vi "fillDataArray.vi"(6 "Data":dbl[][](array[numeric]), 8 "error in (no error)":errorcluster, 9 "fill number":i32[](array[numeric]), 10 "position":i32[](array[numeric]), 11 "SoundAO in":refnum<class "SoundAO.lvclass">) -> (0 "error out":errorcluster, 2 "transformedData":dbl[][](array[numeric]), 3 "SoundAO out":refnum<class "SoundAO.lvclass">)   [LabVIEW 2011, in "Hardware.lvlib" / "Channels.lvlib" / "SoundAO.lvclass"]
uses:
  SoundAO.lvclass
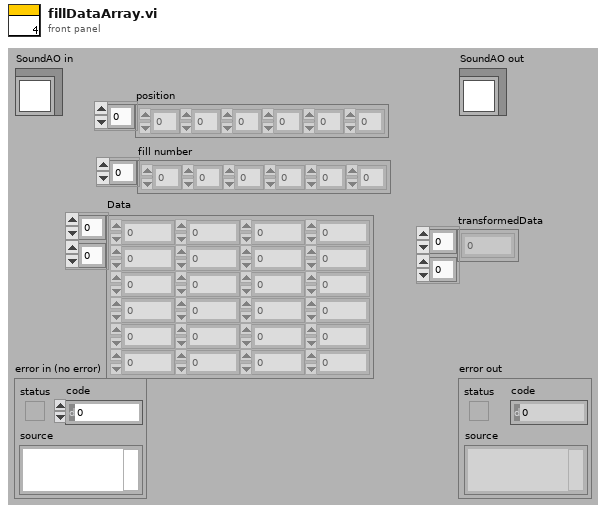
[diagram p1: front panel]
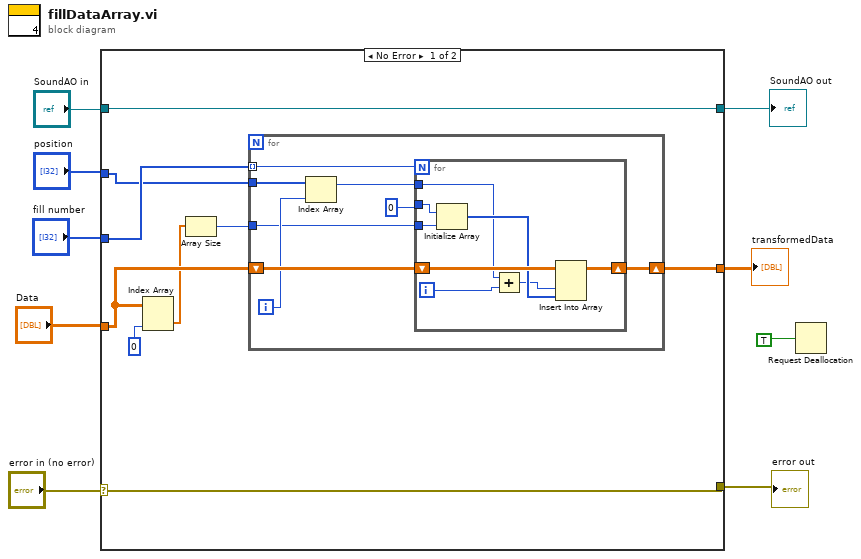
[diagram p0: block diagram]
diagram:
  n1 = case shown="No Error" "error in (no error)" {
    selector: "error in (no error)" -> [w14 w36]
    tunnel: [w14 w36] -> w7
    tunnel: [w16 w35] -> w8
    tunnel: "SoundAO in" -> [w16 w35]
    tunnel: "position" -> [w17 _]
    tunnel: "fill number" -> [w18 _]
    tunnel: "Data" -> [w12 _]
    tunnel: [w13 _] -> w2
    frame No Error {
      n2 = Index Array(array=w12, index (col)=0) -> (element=w10:dbl[])  [unwired: 1 in]
      n3 = Array Size(array=w10) -> (size(s)=w15:i32)
      n4 = for {
        tunnel: w18 -> [w23] mode=indexing
        shift-right: [w24] -> w13
        shift-left: w12 -> [w25]
        tunnel: w17 -> [w22]
        tunnel: w15 -> [w19]
        i -> [w21]
        n5 = Index Array(array=w22, index=w21) -> (element=w20:i32)
        n6 = for {
          N: w23 -> [_]
          tunnel: 0 -> [w34]
          shift-right: [w31] -> w24
          shift-left: w25 -> [w33]
          tunnel: w20 -> [w29]
          tunnel: w19 -> [w27]
          i -> [w30]
          n7 = Initialize Array(w34, w27) -> (w32:i32[])
          n8 = Add(x=w29, y=w30) -> (x+y=w28:i32)
          n9 = Insert Into Array(array=w33, index (col)=w28, new element=w32) -> (w31:dbl[][])  [unwired: 1 in]
        }
      }
    }
    frame Error {
    }
  }
  "error out" <- w7
  "SoundAO out" <- w8
  "transformedData" <- w2
  n10 = Request Deallocation(TRUE) -> ()
